vi "DSF.Engine.Interface.Get Command FIFO.vi"(8 "error in (no error)":errorcluster, 11 "Interface in":refnum<class "DSF.Engine.Interface.lvclass">) -> (0 "error out":errorcluster, 2 "Command FIFO":T1, 3 "Interface out":refnum<class "DSF.Engine.Interface.lvclass">)   [LabVIEW 2016, in "DSF.Engine.lvlib" / "DSF.Engine.Interface.lvclass"]
uses:
  DSF.Engine.Interface.lvclass
  DSF.Engine.Interface.RT FIFO.Ref.16B.ctl
  DSF.Engine.Interface.RT FIFO.Data.16B.ctl
  DSF.Engine.Interface.RT FIFO.Payload.16B.ctl
  DSF.Engine.Interface.lvclass/DSF.Engine.Interface.ctl
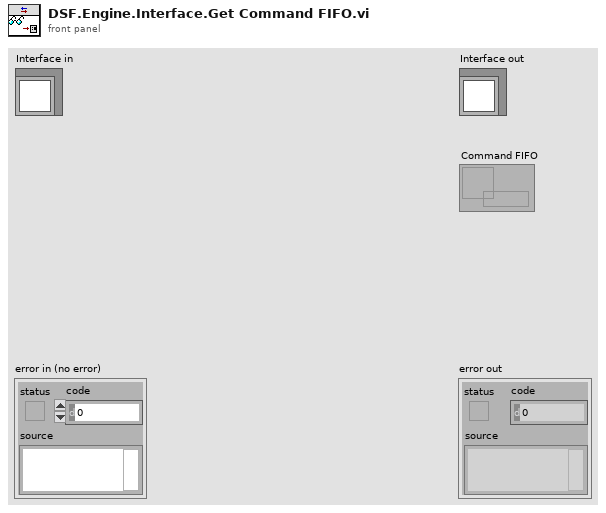
[diagram p1: front panel]
types:
  T1 = typedef "DSF.Engine.lvlib/DSF.Engine.Interface.lvclass/DSF.Engine.Interface.RT FIFO.Ref.16B.ctl" = refnum<k33>
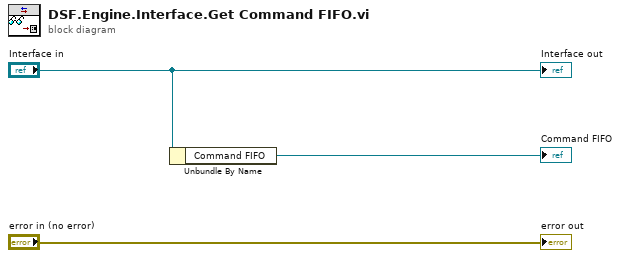
[diagram p0: block diagram]
diagram:
  n1 = Unbundle By Name("Interface in") -> ("Command FIFO"=→"Command FIFO":T1)
  "error out" <- "error in (no error)"
  "Interface out" <- "Interface in"
